vi "Trap_position_vectors.vi"(0 "Data array":u16[](array[numeric])) -> (1 "Output data for plotting":dbl[][](array[numeric]), 2 "Output data for saving":u64[](array[numeric]))   [LabVIEW 2014]
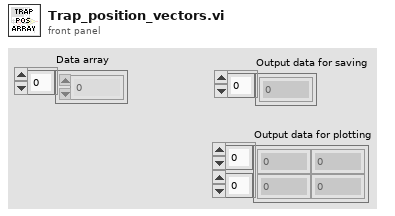
[diagram p1: front panel]
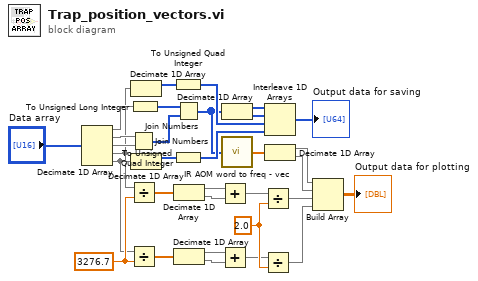
[diagram p0: block diagram]
diagram:
  w20 = 2.0
  w11 = 3276.7
  n1 = Decimate 1D Array("Data array") -> (w30:u16[], w28:u16[], w29:u16[], w9:u16[], w10:u16[])
  n2 = Join Numbers(hi=w28, lo=w29) -> ((hi.lo)=w32:u32[])
  n3 = Divide(x=w9, y=w11) -> (x/y=w12:dbl[])
  n4 = Divide(x=w10, y=w11) -> (x/y=w13:dbl[])
  n5 = To Unsigned Long Integer(number=w30) -> (unsigned 32bit integer=w31:u32[])
  n6 = Decimate 1D Array(w9) -> (w21:u16[])  [unwired: 1 out]
  n7 = Decimate 1D Array(w10) -> (w22:u16[])  [unwired: 1 out]
  n8 = To Unsigned Quad Integer(1:w21) -> (0:w23:u64[])
  n9 = To Unsigned Quad Integer(1:w22) -> (0:w24:u64[])
  n10 = Join Numbers(hi=w31, lo=w32) -> ((hi.lo)=w3:u64[])
  n11 = Decimate 1D Array(w12) -> (w14:dbl[], w15:dbl[])
  n12 = Decimate 1D Array(w13) -> (w16:dbl[], w17:dbl[])
  n13 = Add(x=w14, y=w15) -> (x+y=w18:dbl[])
  n14 = Add(x=w16, y=w17) -> (x+y=w19:dbl[])
  n15 = Decimate 1D Array(w3) -> (w26:u64[], w25:u64[])
  n16 = call "IR AOM word to freq - vec.vi"("Frequency Word In (double vec)"=w3) -> ("Frequency Out"=w6:dbl[])
  n17 = Divide(x=w18, y=w20) -> (x/y=w5:dbl[])
  n18 = Divide(x=w19, y=w20) -> (x/y=w4:dbl[])
  n19 = Interleave 1D Arrays(w26, w25, w23, w24) -> (→"Output data for saving":u64[])
  n20 = Decimate 1D Array(w6) -> (w7:dbl[], w8:dbl[])
  n21 = Build Array(w7, w8, w5, w4) -> (→"Output data for plotting":dbl[][])
